vi "UM2.vi"() -> ()   [LabVIEW 2020]
uses:
  Machine.ctl
  Arrays.ctl
  Array.ctl
  Platter.ctl
panel:
  out "Numeric 2":i32
  out "Array":dbl[](array[numeric])
  out "Numeric":i32
  in  "Path":path=path "/Users/toshi/Documents/UM/codex.umz"
  out "output":string
  out "current machine":T1={"Arrays"={}, "Finger"=0, "Registers"=[], "next id"=1} {"Registers" format="%032b"; "Arrays"."Array" format="%032b"}
  in  "input":string="(\\b.bb)(\\v.vv)06FHPVboundvarHRAk"
  out "read program":T3 format="%032b"
  in  "initial machine state":T1={"Arrays"={}, "Finger"=0, "Registers"=[0, 0, 0, 0, 0, 0, 0, 0], "next id"=1} {"Registers" format="%032b"; "Arrays"."Array" format="%032b"}
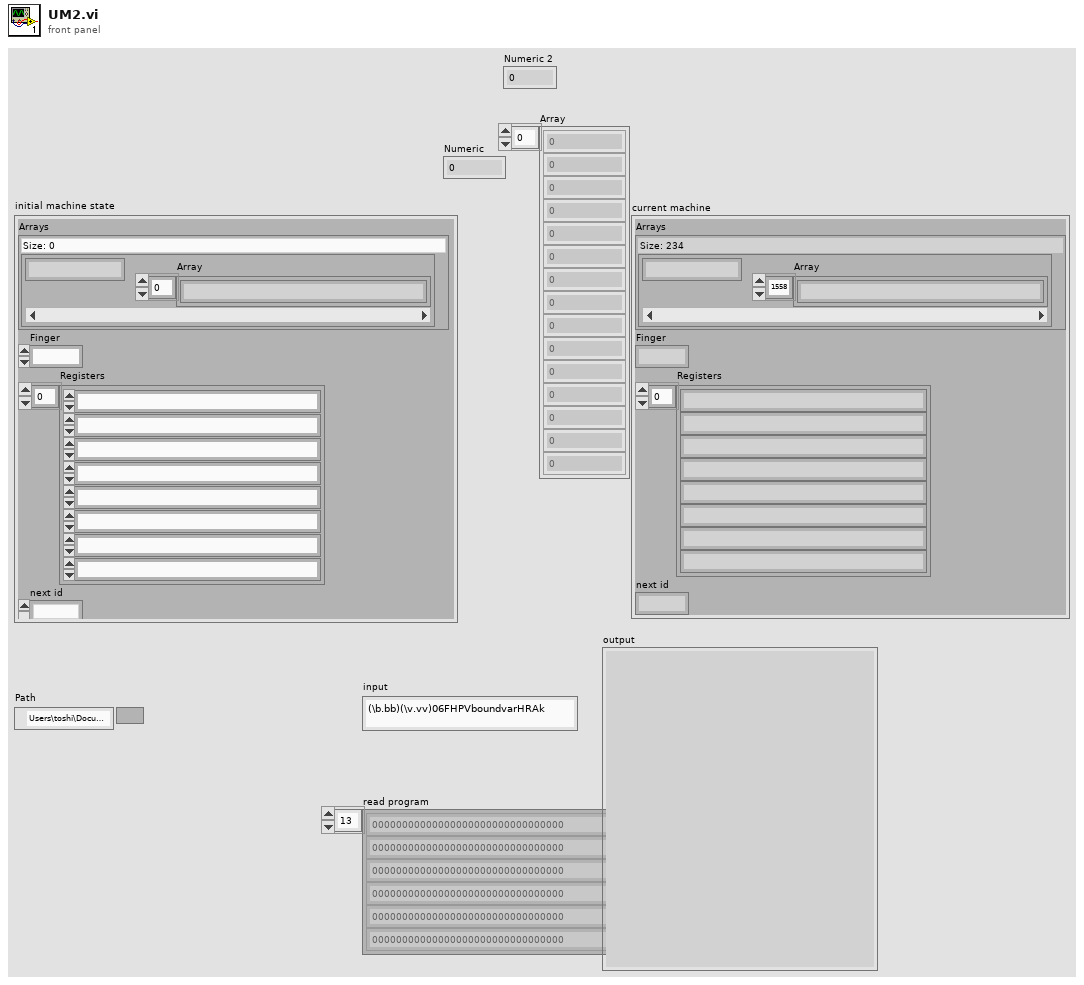
[diagram p1: front panel]
types:
  T1 = typedef "Machine.ctl" = cluster{"Arrays":T2, "Finger":u32, "Registers":T4[], "next id":u32}
  T2 = typedef "Arrays.ctl" = map{string, T3}
  T3 = typedef "Array.ctl" = T4[]
  T4 = typedef "Platter.ctl" = u32
  T5 = enum16{"big-endian, network order", "native, host order", "little-endian"}
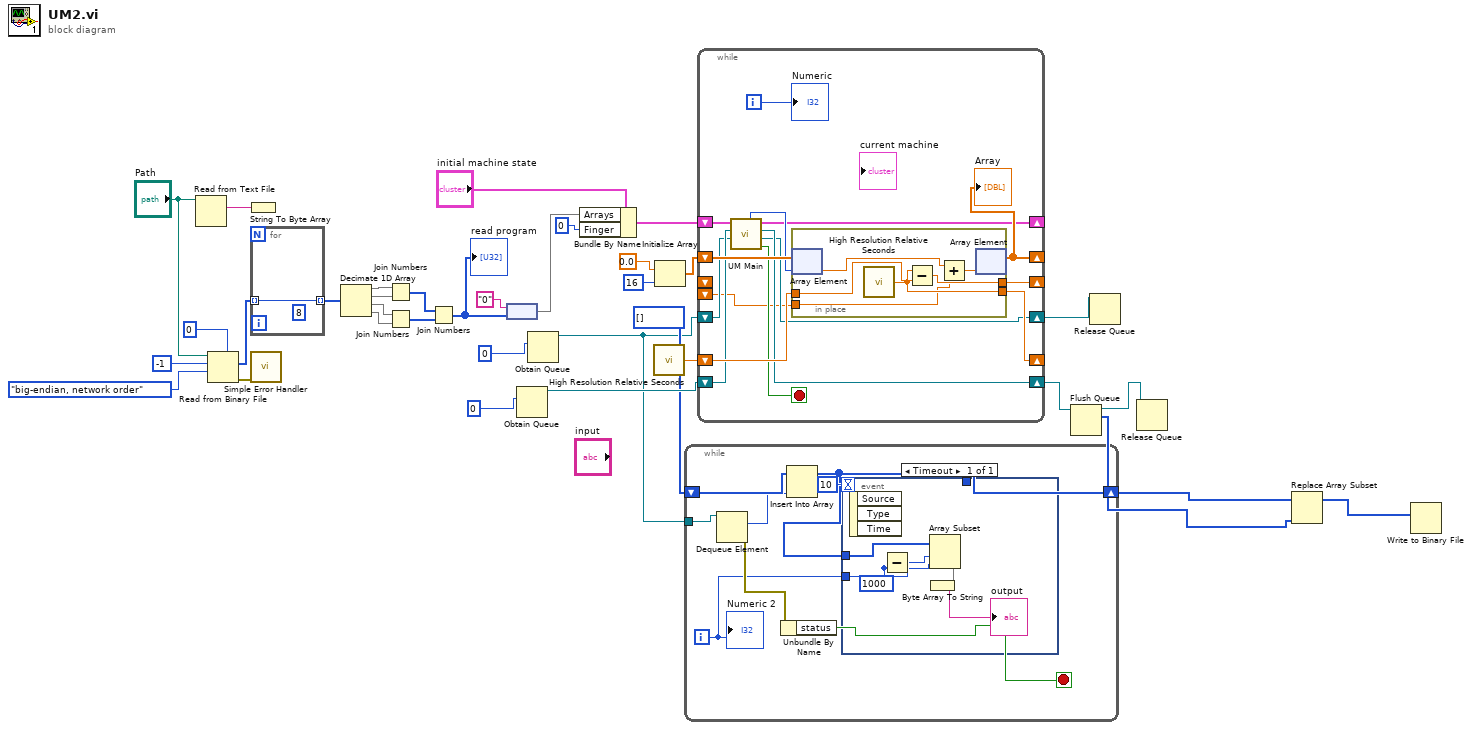
[diagram p0: block diagram]
diagram:
  n1 = Read from Text File(file (use dialog)="Path") -> (text=w21:string)  [unwired: 3 in, 3 out]
  n2 = Read from Binary File(5:u8 0, 9:T5."big-endian, network order" ("byte order (0:big-endian, network order)"), 10:-1 ("count (1)"), 11:"Path") -> (0:w23:errorcluster, 2:w18:u8[])  [unwired: 2 in, 2 out]
  n3 = String To Byte Array(string=w21) -> ()  [unwired: 1 out]
  n4 = for {
    tunnel: w18 -> [w36] mode=indexing
    tunnel: [w36] -> w17 mode=indexing
    (unwired) 8
  }
  n5 = call <vilib>:"Simple Error Handler.vi"("error in (no error)"=w23) -> ()  [unwired: 4 in, 5 out]
  n6 = Decimate 1D Array(w17) -> (w30:u8[], w31:u8[], w32:u8[], w33:u8[])
  n7 = Join Numbers(hi=w30, lo=w31) -> ((hi.lo)=w34:u16[])
  n8 = Join Numbers(hi=w32, lo=w33) -> ((hi.lo)=w35:u16[])
  n9 = Join Numbers(hi=w34, lo=w35) -> ((hi.lo)=w28:u32[])
  "read program" <- w28
  n10 = node("0" ("key"), w28) -> (w27:map{string, u32[]})
  n11 = Obtain Queue(element data type=u8 0) -> (queue out=w10:refnum<queue>)  [unwired: 4 in, 2 out]
  n12 = Obtain Queue(element data type=u8 0) -> (queue out=w6:refnum<queue>)  [unwired: 4 in, 2 out]
  n13 = Bundle By Name(cluster="initial machine state", "Arrays"=w27, "Finger"=u32 0) -> (w24:T1)
  n14 = call <vilib>:"High Resolution Relative Seconds.vi"() -> ("relative seconds"=w12:dbl)
  n15 = Initialize Array(0.0 ("element"), 16 ("dimension size")) -> (w13:dbl[])
  n16 = while {
    shift-right: [w37] -> w3
    shift-left: u8[] [] -> [w44]
    tunnel: w6 -> [w43]
    i -> [w38]
    stop <- w40 stop-if-true
    n17 = Dequeue Element(queue=w43) -> (element=w42:u8, error out=w41:errorcluster)  [unwired: 2 in, 2 out]
    n18 = Unbundle By Name(w41) -> ("status"=w40:bool)
    n19 = Insert Into Array(array=w44, new element=w42) -> (w37:u8[])  [unwired: 1 in]
    n20 = event shown="[0] Timeout" {
      selector: _ -> [_]
      dyn-events: _ -> [_]
      timeout: 10 -> [_]
      tunnel: w37 -> [w50]
      tunnel: w38 -> [w49]
      tunnel: w37 -> [_]
      event Timeout {
        w47 = 1000 ("y")
        n21 = event-data() -> ()  [unwired: 1 in, 3 out]
        n22 = Subtract(x=w49, y=w47) -> (x-y=w48:i32)
        n23 = Array Subset(array=w50, index=w48, length=w47) -> (w46:u8[])
        n24 = Byte Array To String(unsigned byte array=w46) -> (string=→"output":string)
      }
    }
    "Numeric 2" <- w38
  }
  n25 = while {
    shift-right: [w51] -> _
    shift-left: w24 -> [w61]
    shift-right: [w55] -> w7
    shift-left: w6 -> [w59]
    shift-right: [w57] -> w5
    shift-left: w10 -> [w60]
    shift-right: [w54] -> _
    shift-left: w13 -> [w64]
    shift-right: [w62] -> _
    shift-left: w12 -> [w63]
    shift-right: [w53] -> _
    shift-left: _ -> [_]
    shift-left: _ -> [w52]
    i -> [w65]
    stop <- w56 stop-if-true
    n26 = call "UM Main.vi"("output in"=w59, "input in"=w60, "machine in"=w61) -> ("terminate"=w56:bool, "output out"=w55:refnum<queue>, "input out"=w57:refnum<queue>, "machine out"=w51:T1, "instruction out"=w58:T4)  [unwired: 2 in]
    n27 = in-place {
      in-place-border: w63 -> [w70]
      in-place-border: [w68] -> w62
      in-place-border: [w67] -> w53
      in-place-border: w52 -> [w66]
      n28 = in-place-array #1(w64, w58) -> (w69:dbl)
      n29 = call <vilib>:"High Resolution Relative Seconds.vi"() -> ("relative seconds"=w68:dbl)
      n30 = Subtract(x=w68, y=w70) -> (x-y=w67:dbl)
      n31 = Add(x=w69, y=w66) -> (x+y=w71:dbl)
      n32 = in-place-array #1(w71) -> (w54:dbl[])  [unwired: 1 out]
    }
    "Array" <- w54
    "Numeric" <- w65
  }
  n33 = Flush Queue(queue=w5) -> (queue out=w4:refnum<queue>, remaining elements=w2:u8[])  [unwired: 1 in, 1 out]
  n34 = Release Queue(queue=w7) -> ()  [unwired: 2 in, 3 out]
  n35 = Release Queue(queue=w4) -> ()  [unwired: 2 in, 3 out]
  n36 = Replace Array Subset(array=w3, new element=w2) -> (w1:u8[])  [unwired: 1 in]
  n37 = Write to Binary File(data=w1) -> ()  [unwired: 5 in, 3 out]
